vi "IR Scan2.vi"() -> ()   [LabVIEW 2013]
uses:
  <vilib>/Platform/TimedLoop/XDataNode/timing_clust.ctl
  <vilib>/Platform/TimedLoop/XDataNode/nitl_modes.ctl
  <vilib>/Platform/TimedLoop/XDataNode/wakeup.ctl
  <vilib>/robotics/Obstacle Avoidance/Simple Vector Field Histogram/Panic Range.ctl
  <vilib>/FPGAPlugInAG/sbRIO-9642/niLvFpga_Open_sbRIO-9642.vi
  <vilib>/rvi/interface/common/dynamic/niFpgaDynamicAddResources.vi
  <vilib>/Utility/AngleManip/Degrees to Radians (Scalar DBL).vi
  <vilib>/rvi/interface/common/niFpgaWaitOnOcc.vi
  <vilib>/Utility/error.llb/Error Cluster From Error Code.vi
  <vilib>/rvi/errors/niLvFpgaAdjustHostInterfaceError.vi
  <vilib>/Platform/TimedLoop/XDataNode/XDataNode.xnode
  <vilib>/rvi/interface/nirviOpenFPGA/nirviOpenFPGA.xnode
  FPGA Bitfiles/NatesProject1_FPGATarget_FPGAConfig_gDHlPw7zMRU.lvbitx
  FPGA Config.vi
  <vilib>/rvi/interface/nirviReadWriteControl/nirviReadWriteControl.xnode
  <vilib>/robotics/Utilities/Scan Angles/NI_Robotics_Scan Angles.lvlib
  <vilib>/Platform/TimedLoop/XDataNode/XDNodeRunTimeDep.lvlib
  <vilib>/robotics/Obstacle Avoidance/Simple Vector Field Histogram/NI_Robotics_Simple Vector Field Histogram.lvlib
  <vilib>/Utility/AngleManip/NI_AngleManipulation.lvlib
  NiFpgaLv.dll
  <vilib>/rvi/interface/Simulation/niFpgaSimulationCallBeginRW.vi
panel:
  out "angle to obstacle":dbl
  out "distance to obstacle":dbl
  out "size of gap":dbl
  out "angle to gap":dbl
  out "Sensor Data":cluster{"angles (deg)":dbl[], "distances":dbl[]}(graph)
  out "Front Sensor\nDistance\n(cm)":dbl(slide) scale=0.0..150.0
  in  "stop":bool
  out "ModA/AI0":fxp<+/-,26,5>
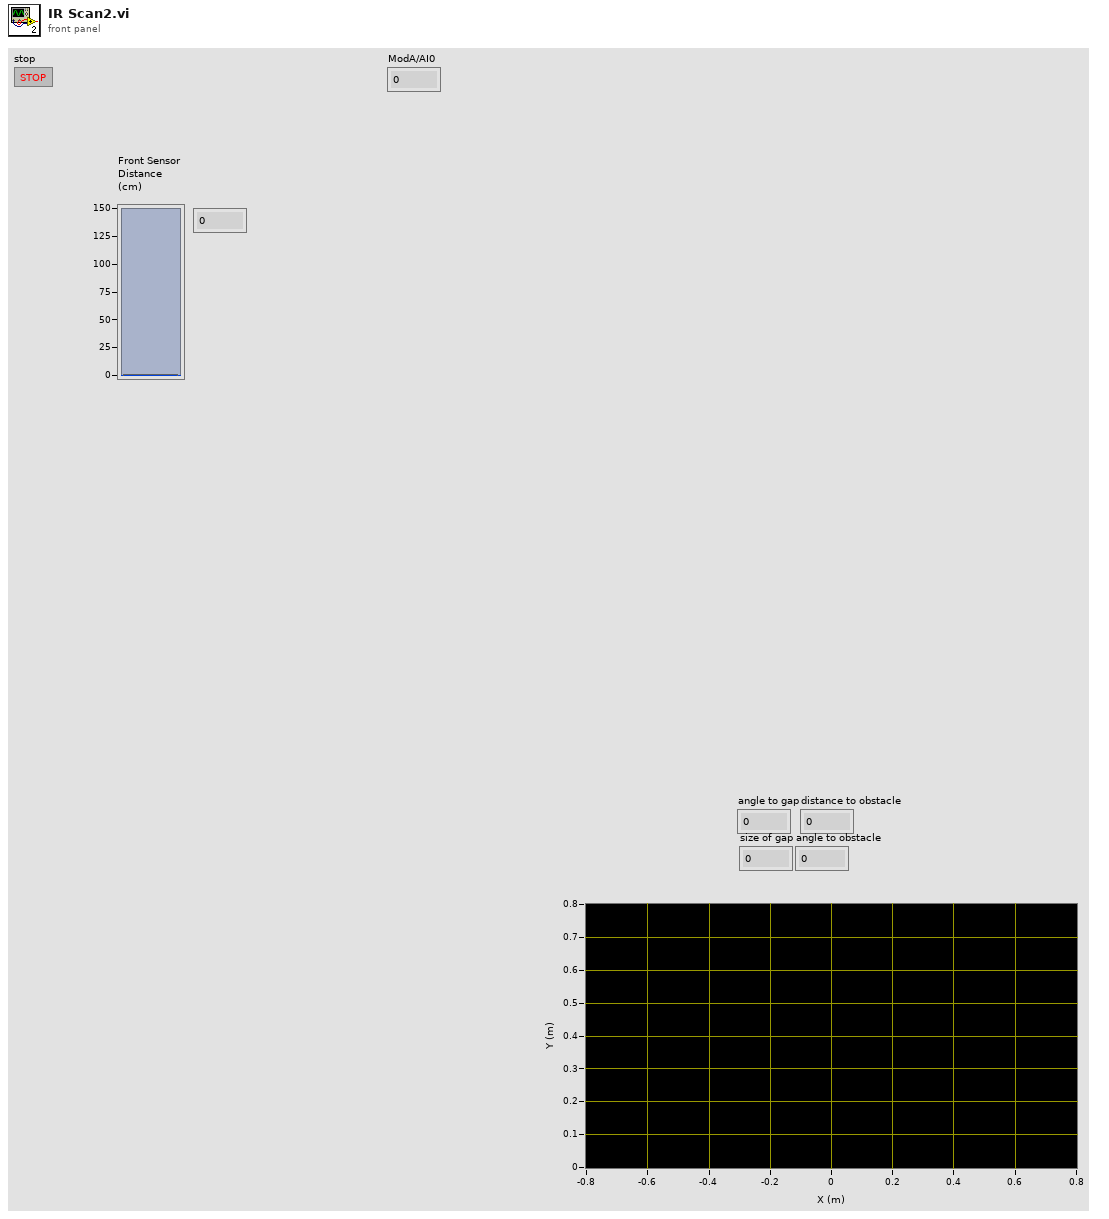
[diagram p1: front panel]
types:
  T1 = typedef "NI_Robotics_Scan Angles.lvlib/Scan Angle Data.ctl" = cluster{"angles":dbl[], "distances":dbl[], "current index":i32, "previous index":i32}
  T2 = typedef "XDNodeRunTimeDep.lvlib/timing_clust.ctl" = cluster{"Expected End [f-1]":u64, "Actual End [f-1]":u64, "Finished Late? [f-1]":bool, "Expected End [i-1]":u64, "Actual End [i-1]":u64, "Finished Late? [i-1]":bool, "Expected Start [i]":u64, "Actual Start [i]":u64, "Expected Start [f]":u64, "Actual Start [f]":u64, "Source Name":string, "Structure Name":string, "Period":i64, "Deadline":i64, "Offset":i64, "Start":i64, "Priority":i32, "Timeout":i32, "Mode":T3, "Wakeup Reason":T4, "Error":errorcluster, "Source Type":string, "Secondary Source Type":string, "Global End Time":u64, "Global Start Time":u64, "Frame Duration":u64, "Iteration Duration":u64, "Assigned CPU":i32, "I/O Scan Engine Mode":u32}
  T3 = typedef "XDNodeRunTimeDep.lvlib/nitl_modes.ctl" = enum32{"No Change", "Process missed periods, maintain original phase", "Discard missed periods, maintain original phase", "Process missed periods, ignore original phase", "Discard missed periods, ignore original phase"}
  T4 = typedef "XDNodeRunTimeDep.lvlib/wakeup.ctl" = enum32{"Normal", "Aborted", "Asynchronous wakeup", "Timing source error", "Timed loop error", "Timeout"}
  T5 = typedef "NI_Robotics_Simple Vector Field Histogram.lvlib/Panic Range.ctl" = cluster{"panic threshold distance (0)":dbl, "panic threshold angle (0)":dbl}
  T6 = typedef "NI_Robotics_Simple Vector Field Histogram.lvlib/Obstacle Description.ctl" = cluster{"angle to obstacle":dbl, "distance to obstacle":dbl}
  T7 = typedef "NI_Robotics_Simple Vector Field Histogram.lvlib/Gap Description.ctl" = cluster{"angle to gap":dbl, "size of gap":dbl}
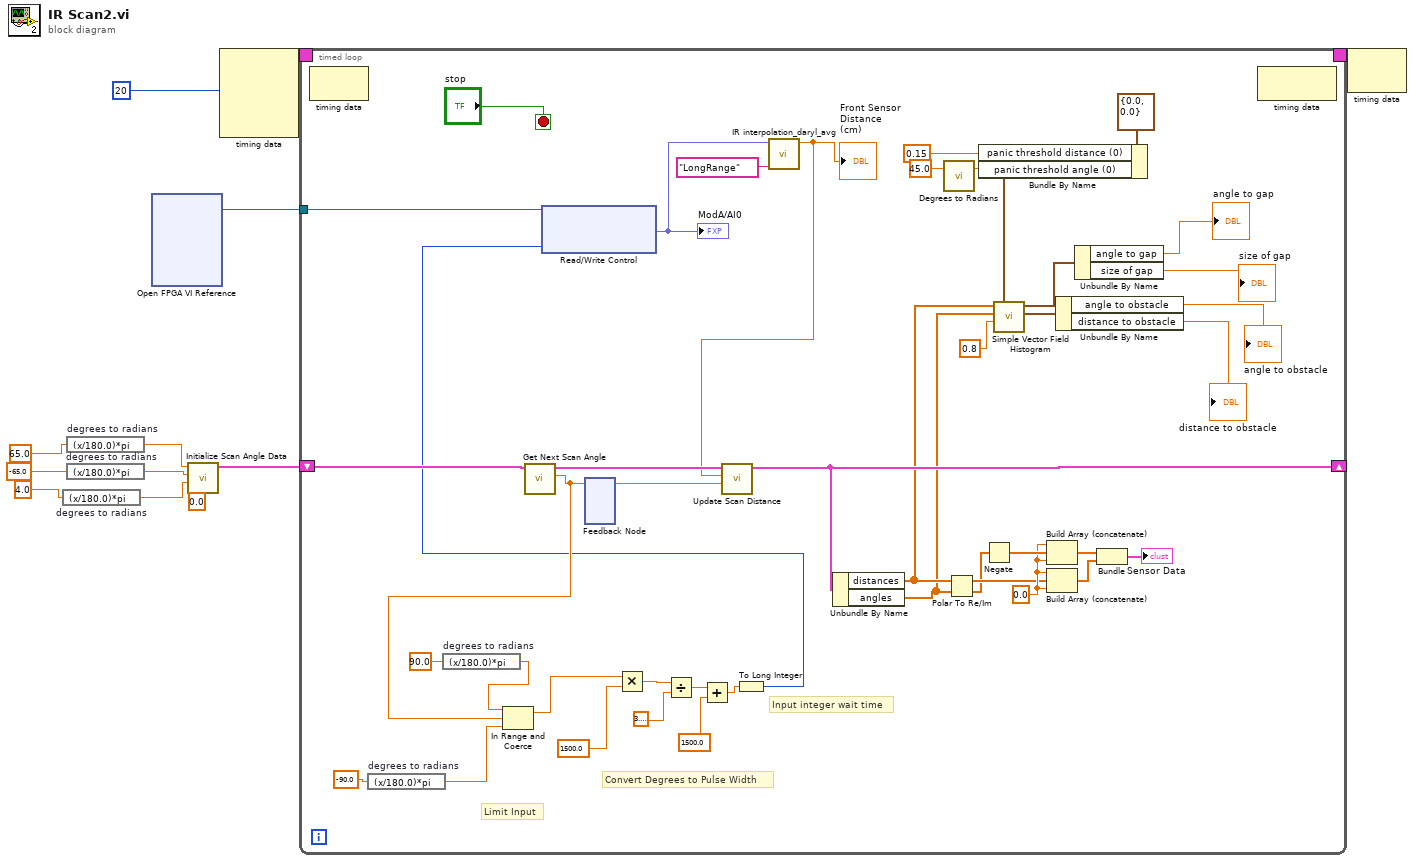
[diagram p0: block diagram]
diagram:
  n1 = expression code="(x/180.0)*pi" "degrees to radians"(4.0 ("scan angle")) -> (w3:dbl)
  n2 = expression code="(x/180.0)*pi" "degrees to radians"(65.0 ("max angle")) -> (w5:dbl)
  n3 = expression code="(x/180.0)*pi" "degrees to radians"(-65.0 ("min angle")) -> (w4:dbl)
  n4 = xnode "Open FPGA VI Reference"() -> ("FPGA VI Reference Out"=w12:refnum<k20>)  [unwired: 2 in, 1 out]
  n5 = call <vilib>:"Initialize Scan Angle Data.vi"("initial angle (0)"=0.0, "scan angle"=w3, "min angle"=w4, "max angle"=w5) -> ("scan angles"=w10:T1)  [unwired: 6 in, 1 out]
  n6 = node-c288(i64 20 ("Period")) -> (w9:T2)  [unwired: 3 in]
  n7 = timed-loop {
    tunnel: w12 -> [w52]
    shift-right: [w27] -> _
    shift-left: w10 -> [w49]
    timing: w9 -> [_]
    timing-out: [_] -> w8
    stop <- "stop" stop-if-true
    w32 = 0.0 ("element")
    # "Input integer wait time"
    # "Convert Degrees to Pulse Width"
    # "Limit Input"
    n8 = node-c288() -> ()  [unwired: 1 in, 1 out]
    n9 = expression code="(x/180.0)*pi" "degrees to radians"(-90.0 ("lower limit")) -> (w36:dbl)
    n10 = expression code="(x/180.0)*pi" "degrees to radians"(90.0 ("upper limit")) -> (w35:dbl)
    n11 = call <vilib>:"Get Next Scan Angle.vi"("scan angles in"=w49) -> ("new angle"=w41:dbl, "scan angles out"=w51:T1)  [unwired: 9 in]
    n12 = In Range and Coerce(upper limit=w35, x=w41, lower limit=w36) -> (coerced(x)=w47:dbl)  [unwired: 1 out]
    n13 = feedback #1() -> (w50:dbl)  [unwired: 1 in]
    n14 = feedback-in #1(w41) -> ()
    n15 = Multiply(x=w47, y=1500.0) -> (x*y=w46:dbl)
    n16 = Divide(x=w46, y=3.141592653589793) -> (x/y=w44:dbl)
    n17 = Add(x=w44, y=1500.0) -> (x+y=w43:dbl)
    n18 = To Long Integer(number=w43) -> (32bit integer=w40:i32)
    n19 = xnode "Read/Write Control"("FPGA VI Reference In"=w52, "Pulse Width(uSec)"=w40) -> ("ModA/AI1"=w54:fxp<+/-,26,5>)  [unwired: 1 in, 2 out]
    "ModA/AI0" <- w54
    n20 = call "IR interpolation_daryl_avg.vi"("IR Sensor Type"="LongRange", "x value"=w54) -> ("interpolation value"=w48:dbl)  [unwired: 9 in]
    "Front Sensor\nDistance\n(cm)" <- w48
    n21 = call <vilib>:"Update Scan Distance.vi"("scan angle"=w50, "new scan distance"=w48, "scan angles in"=w51) -> ("scan angles out"=w27:T1)  [unwired: 8 in]
    n22 = Unbundle By Name(w27) -> ("distances"=w26:dbl[], "angles"=w25:dbl[])
    n23 = call-poly <vilib>:"Degrees to Radians.vi"("angle (deg)"=45.0 ("panic threshold angle (rad)")) -> ("angle (rad)"=w17:dbl)  [unwired: 2 in]
    n24 = Polar To Re/Im(2:w25, 3:w26) -> (0:w29:dbl[], 1:w30:dbl[])
    n25 = Bundle By Name(cluster=T5 {"panic threshold distance (0)"=0.0, "panic threshold angle (0)"=0.0} ("panic range"), "panic threshold distance (0)"=0.15 ("panic threshold distance (m)"), "panic threshold angle (0)"=w17) -> (w13:T5)
    n26 = Negate(x=w29) -> (-x=w34:dbl[])
    n27 = call <vilib>:"Simple Vector Field Histogram.vi"("panic range"=w13, "distance threshold"=0.8, "direction angles"=w25, "distances"=w26) -> ("nearest obstacle"=w23:T6, "largest gap"=w22:T7)  [unwired: 3 in, 3 out]
    n28 = Build Array (concatenate)(w32, w34, w32) -> (w33:dbl[])
    n29 = Build Array (concatenate)(w32, w30, w32) -> (w31:dbl[])
    n30 = Unbundle By Name(w23) -> ("angle to obstacle"=→"angle to obstacle":dbl, "distance to obstacle"=→"distance to obstacle":dbl)
    n31 = Unbundle By Name(w22) -> ("angle to gap"=→"angle to gap":dbl, "size of gap"=→"size of gap":dbl)
    n32 = Bundle(w33, w31) -> (→"Sensor Data":cluster{dbl[], dbl[]})  [unwired: 1 in]
    n33 = node-c288() -> ()  [unwired: 1 in, 1 out]
  }
  n34 = node-c288(w8) -> ()  [unwired: 1 out]
